vi "Executing.vi"(8 "error in (no error)":errorcluster, 11 "Command in":refnum<class "Do Nothing.lvclass">) -> (0 "error out":errorcluster, 3 "Command out":refnum<class "Do Nothing.lvclass">)   [LabVIEW 2013, in "Receiver.lvlib" / "Receive Commands Using State Actors.lvlib" / "Do Nothing.lvlib" / "Do Nothing.lvclass"]
uses:
  Do Nothing.lvclass
  Receiver Command.lvclass
  <vilib>/ActorFramework/Actor/Actor.lvclass/Actor.ctl
  <vilib>/ActorFramework/Message Enqueuer/Message Enqueuer.lvclass/Message Enqueuer.ctl
  <vilib>/ActorFramework/Message Enqueuer/Init from Existing Queue.vi
  <vilib>/ActorFramework/Message Enqueuer/Enqueue.vi
  <vilib>/ActorFramework/Message Priority Queue/Priority Enqueue.vi
  <vilib>/ActorFramework/Message Enqueuer/Message Enqueuer.lvclass
  Command State Actor Messages/Go To Completing Msg/Go To Completing Msg.lvclass
  <vilib>/ActorFramework/Actor/Actor.lvclass
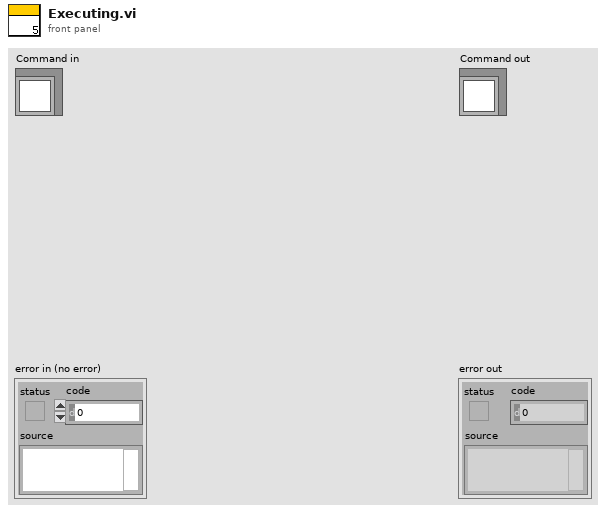
[diagram p1: front panel]
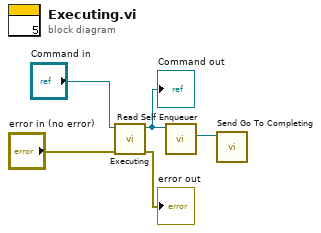
[diagram p0: block diagram]
diagram:
  n1 = call-parent "Executing.vi"("error in (no error)"="error in (no error)", "Command in"="Command in") -> ("error out"=→"error out":errorcluster, "Command out"=w2:refnum<class "Do Nothing.lvclass">)  [unwired: 8 in]
  "Command out" <- w2
  n2 = call <vilib>:"Read Self Enqueuer.vi"("Actor"=w2) -> ("Self Enqueuer"=w1:refnum<class "Message Enqueuer.lvclass">)  [unwired: 10 in]
  n3 = call "Send Go To Completing.vi"("Message Enqueuer"=w1) -> ()  [unwired: 9 in, 2 out]
